vi "output.vi"(8 "error in":errorcluster, 10 "data table in":T1, 11 "SystemLin Tag Module runtime in":refnum<class "SystemLink runtime.lvclass">) -> (0 "error out":errorcluster, 2 "data table out":T1, 3 "SystemLin Tag Module runtime out":refnum<class "SystemLink runtime.lvclass">)   [LabVIEW 2014, in "SystemLink runtime.lvclass"]
doc: "Provides an interface for writing data to a module at runtime. While this interface performs no operations, a child should provide an override which may write to any open sessions, references, or interfaces."
uses:
  SystemLink runtime.lvclass
  <vilib>/NI/Tag Bus/table/data table.ctl
  SystemLink runtime.lvclass/SystemLink runtime.ctl
  <vilib>/NI/Tag Bus/table/data polymorphs/read one/read Double.vi
  <vilib>/NI/Tag Bus/table/data polymorphs/read one/read Single.vi
  <vilib>/NI/Tag Bus/table/data polymorphs/read one/read I32.vi
  <vilib>/NI/Tag Bus/table/data polymorphs/read one/read I16.vi
  <vilib>/NI/Tag Bus/table/data polymorphs/read one/read I8.vi
  <vilib>/NI/Tag Bus/table/data polymorphs/read one/read Boolean.vi
  <vilib>/NI/Tag Bus/table/data polymorphs/read one/read String.vi
  <vilib>/NI/Tag Bus/table/data table.lvlib
  <vilib>/Skyline/Tag/Wrapper/Wrapper_class/NI Skyline Tag.lvclass
  <vilib>/Skyline/Tag/Wrapper/Wrapper_class/Write Tag (DBL).vi
  <vilib>/Skyline/Tag/Wrapper/Wrapper_class/Write Tag (I32).vi
  <vilib>/Skyline/Tag/Wrapper/Wrapper_class/Write Tag (String).vi
  <vilib>/Skyline/Tag/Wrapper/Wrapper AMQP_class/NI Skyline Tag AMQP.lvclass
  <vilib>/Skyline/Tag/Wrapper/Wrapper HTTP_class/NI Skyline Tag HTTP.lvclass
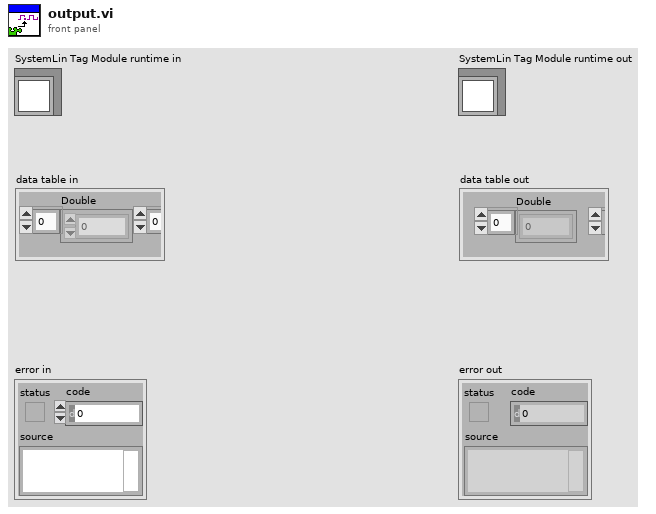
[diagram p1: front panel]
types:
  T1 = typedef "tag bus.lvlib/data table.lvlib/data table.ctl" = cluster{"Double":dbl[], "Single":sgl[], "I64":i64[], "I32":i32[], "I16":i16[], "I8":i8[], "U64":u64[], "U32":u32[], "U16":u16[], "U8":u8[], "Boolean":bool[], "String":string[], "Array of Double":cluster{"DBL Array":dbl[]}[], "Array of Single":cluster{"SGL Array":sgl[]}[], "Array of I64":cluster{"I64 Array":i64[]}[], "Array of I32":cluster{"I32 Array":i32[]}[], "Array of I16":cluster{"I16 Array":i16[]}[], "Array of I8":cluster{"I8 Array":i8[]}[], "Array of U64":cluster{"U64 Array":u64[]}[], "Array of U32":cluster{"U32 Array":u32[]}[], "Array of U16":cluster{"U16 Array":u16[]}[], "Array of U8":cluster{"U8 Array":u8[]}[], "Array of Boolean":cluster{"Boolean Array":bool[]}[], "Array of String":cluster{"String Array":string[]}[]}
  T2 = typedef "SystemLink configuration.lvclass/SysLink Mapping.ctl" = cluster{"Data Type":T3, "Tag Reference":refnum<class "NI Skyline Tag.lvclass">, "Tag Bus Index":i32, "AMQP":bool, "Skylink Index":i32}
  T3 = typedef "tag bus.lvlib/tag descriptor.lvclass/Data Type.ctl" = enum16{"Double", "Single", "I64", "I32", "I16", "I8", "U64", "U32", "U16", "U8", "Boolean", "String", "Array of Double", "Array of Single", "Array of I64", "Array of I32", "Array of I16", "Array of I8", "Array of U64", "Array of U32", "Array of U16", "Array of U8", "Array of Boolean", "Array of String"}
  T4 = typedef "NI Skyline Tag.lvlib/Tag Cluster Wrapper.ctl" = cluster{"Configuration":refnum<class "NI Skyline Configuration.lvclass">, "Tag Cluster":T5}
  T5 = typedef "NI Skyline Tag.lvlib/Tag Cluster.ctl" = cluster{"Path":string, "Data Type":T6, "Value":variant, "Time Stamp":timestamp}
  T6 = typedef "NI Skyline Tag.lvlib/DataType.ctl" = enum32{"Double", "Integer", "String"}
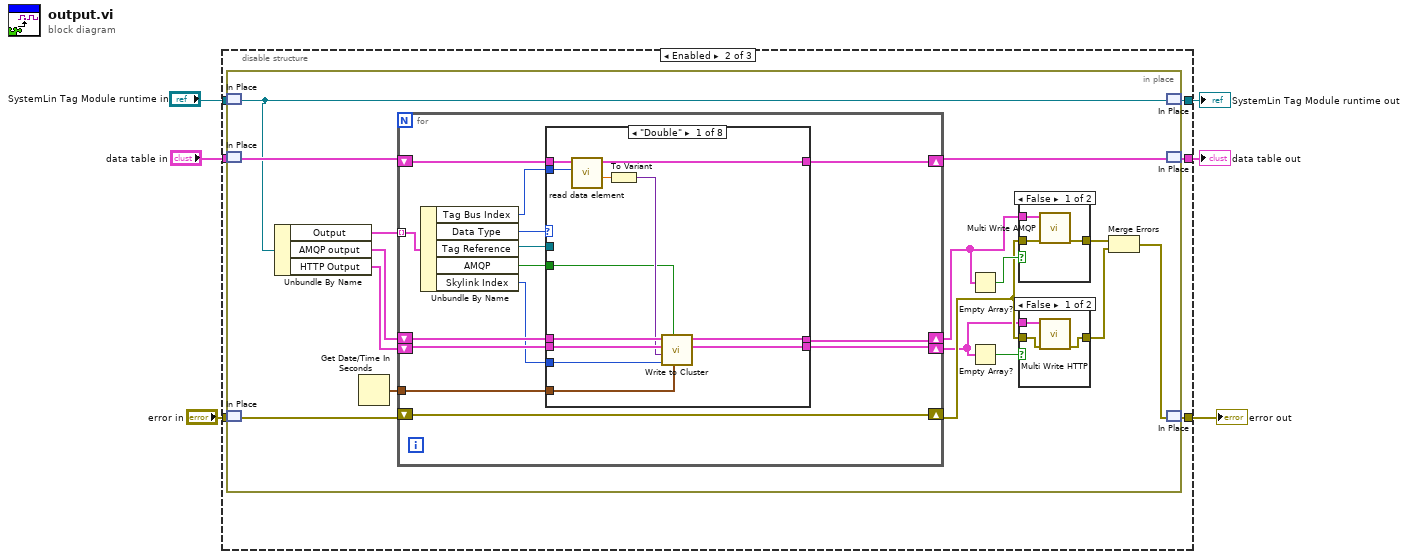
[diagram p0: block diagram]
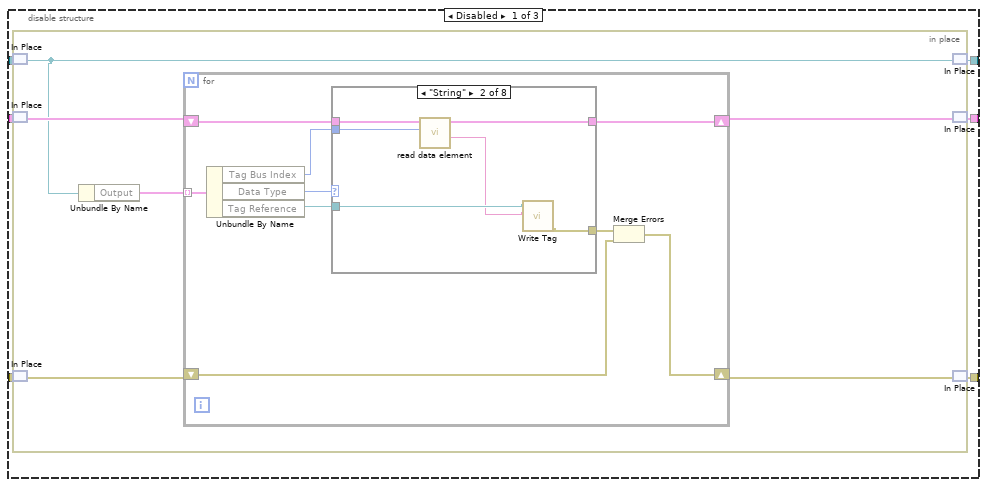
[diagram p2: hidden frame]
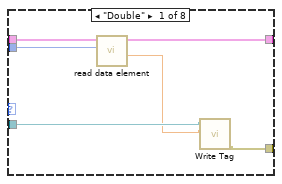
[diagram p3: hidden frame]
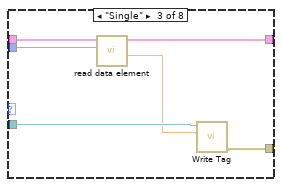
[diagram p4: hidden frame]
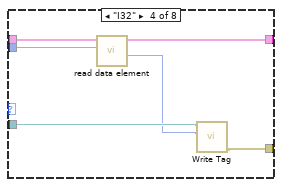
[diagram p5: hidden frame]
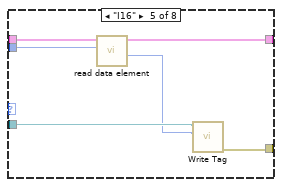
[diagram p6: hidden frame]
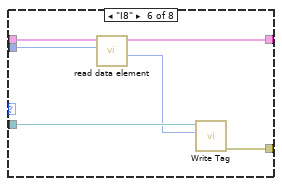
[diagram p7: hidden frame]
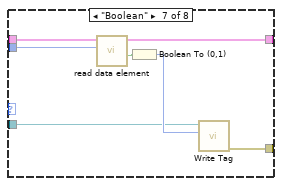
[diagram p8: hidden frame]
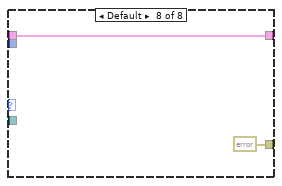
[diagram p9: hidden frame]
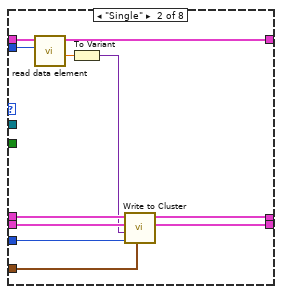
[diagram p12: hidden frame]
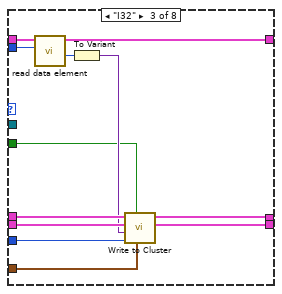
[diagram p13: hidden frame]
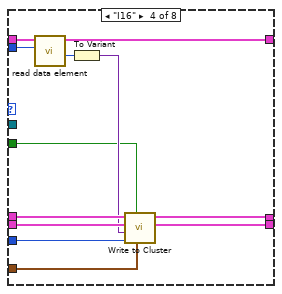
[diagram p14: hidden frame]
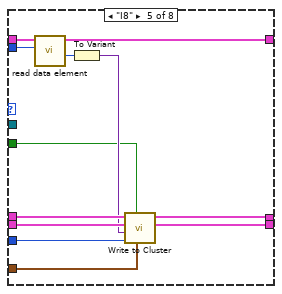
[diagram p15: hidden frame]
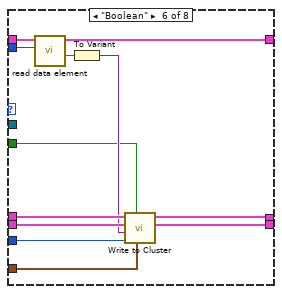
[diagram p16: hidden frame]
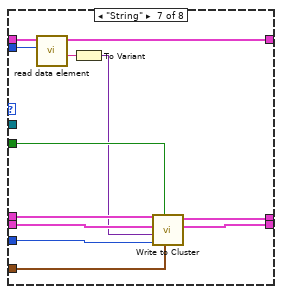
[diagram p17: hidden frame]
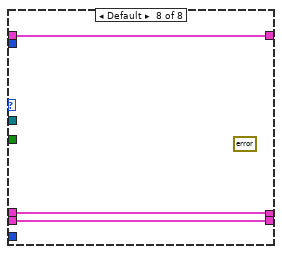
[diagram p18: hidden frame]
diagram:
  n1 = disable-structure shown="Enabled" {
    disable-tunnel: "SystemLin Tag Module runtime in" -> [w12 w78 _]
    disable-tunnel: [w11 w77 _] -> w5
    disable-tunnel: [w10 w76 _] -> w4
    disable-tunnel: [w9 w75 _] -> w3
    disable-tunnel: "data table in" -> [w8 w74 _]
    disable-tunnel: "error in" -> [w7 w73 _]
    frame Disabled {
      n2 = in-place {
        n3 = in-place-match #1(w12) -> (w16:refnum<class "SystemLink runtime.lvclass">)
        n4 = in-place-match #2(w8) -> (w18:T1)
        n5 = in-place-match #3(w7) -> (w14:errorcluster)
        n6 = Unbundle By Name(w16) -> ("Output"=w15:T2[])
        n7 = for {
          shift-right: [w24] -> w17
          shift-left: w18 -> [w25]
          tunnel: w15 -> [w27] mode=indexing
          shift-right: [w19] -> w13
          shift-left: w14 -> [w20]
          n8 = Unbundle By Name(w27) -> ("Tag Bus Index"=w22:i32, "Data Type"=w26:T3, "Tag Reference"=w23:refnum<class "NI Skyline Tag.lvclass">)
          n9 = case shown="\"String\"" w26 {
            tunnel: w25 -> [w33 w39 w45 w51 w57 w63 w70 w72]
            tunnel: [w31 w37 w43 w49 w55 w61 w68 w72] -> w24
            tunnel: w23 -> [w30 w36 w42 w48 w54 w60 w64 _]
            tunnel: [w28 w34 w40 w46 w52 w58 w67 errorcluster {"status"=FALSE, "code"=0, "source"=""} ("error IO")] -> w21
            tunnel: w22 -> [w32 w38 w44 w50 w56 w62 w69 _]
            frame "Double" {
              n10 = call-poly <vilib>:"read data element.vi"("index"=w32, "data table in"=w33) -> ("value"=w29:dbl, "data table out"=w31:T1)  [unwired: 8 in]
              n11 = call-poly <vilib>:"Write Tag.vi"("value"=w29, "tag in"=w30) -> ("error out"=w28:errorcluster)  [unwired: 8 in, 1 out]
            }
            frame "String" {
              n12 = call-poly <vilib>:"read data element.vi"("index"=w38, "data table in"=w39) -> ("value"=w35:string, "data table out"=w37:T1)  [unwired: 8 in]
              n13 = call-poly <vilib>:"Write Tag.vi"("value"=w35, "tag in"=w36) -> ("error out"=w34:errorcluster)  [unwired: 8 in, 1 out]
            }
            frame "Single" {
              n14 = call-poly <vilib>:"read data element.vi"("index"=w44, "data table in"=w45) -> ("value"=w41:sgl, "data table out"=w43:T1)  [unwired: 8 in]
              n15 = call-poly <vilib>:"Write Tag.vi"("value"=w41, "tag in"=w42) -> ("error out"=w40:errorcluster)  [unwired: 8 in, 1 out]
            }
            frame "I32" {
              n16 = call-poly <vilib>:"read data element.vi"("index"=w50, "data table in"=w51) -> ("value"=w47:i32, "data table out"=w49:T1)  [unwired: 8 in]
              n17 = call-poly <vilib>:"Write Tag.vi"("value"=w47, "tag in"=w48) -> ("error out"=w46:errorcluster)  [unwired: 8 in, 1 out]
            }
            frame "I16" {
              n18 = call-poly <vilib>:"read data element.vi"("index"=w56, "data table in"=w57) -> ("value"=w53:i16, "data table out"=w55:T1)  [unwired: 8 in]
              n19 = call-poly <vilib>:"Write Tag.vi"("value"=w53, "tag in"=w54) -> ("error out"=w52:errorcluster)  [unwired: 8 in, 1 out]
            }
            frame "I8" {
              n20 = call-poly <vilib>:"read data element.vi"("index"=w62, "data table in"=w63) -> ("value"=w59:i8, "data table out"=w61:T1)  [unwired: 8 in]
              n21 = call-poly <vilib>:"Write Tag.vi"("value"=w59, "tag in"=w60) -> ("error out"=w58:errorcluster)  [unwired: 8 in, 1 out]
            }
            frame "Boolean" {
              n22 = call-poly <vilib>:"read data element.vi"("index"=w69, "data table in"=w70) -> ("value"=w65:bool, "data table out"=w68:T1)  [unwired: 8 in]
              n23 = Boolean To (0,1)(Boolean=w65) -> (0, 1=w66:i16)
              n24 = call-poly <vilib>:"Write Tag.vi"("value"=w66, "tag in"=w64) -> ("error out"=w67:errorcluster)  [unwired: 8 in, 1 out]
            }
            frame Default {
            }
          }
          n25 = Merge Errors(w21, w20) -> (w19:errorcluster)
        }
        n26 = in-place-match #1(w16) -> (w11:refnum<class "SystemLink runtime.lvclass">)
        n27 = in-place-match #2(w17) -> (w10:T1)
        n28 = in-place-match #3(w13) -> (w9:errorcluster)
      }
    }
    frame Enabled {
      n29 = in-place {
        n30 = in-place-match #4(w78) -> (w92:refnum<class "SystemLink runtime.lvclass">)
        n31 = in-place-match #5(w74) -> (w94:T1)
        n32 = in-place-match #6(w73) -> (w90:errorcluster)
        n33 = Unbundle By Name(w92) -> ("Output"=w91:T2[], "AMQP output"=w89:T4[], "HTTP Output"=w88:T4[])
        n34 = Get Date/Time In Seconds() -> (seconds since 1Jan1904=w79:timestamp)
        n35 = for {
          shift-right: [w113] -> w93
          shift-left: w94 -> [w114]
          tunnel: w91 -> [w116] mode=indexing
          shift-right: [w110] -> w83
          shift-left: w90 -> [w110]
          shift-right: [w104] -> w81
          shift-left: w88 -> [w108]
          shift-right: [w105] -> w80
          shift-left: w89 -> [w109]
          tunnel: w79 -> [w103]
          n36 = Unbundle By Name(w116) -> ("Tag Bus Index"=w111:i32, "Data Type"=w115:T3, "Tag Reference"=w112:refnum<class "NI Skyline Tag.lvclass">, "AMQP"=w107:bool, "Skylink Index"=w106:i32)
          n37 = case shown="\"Double\"" w115 {
            tunnel: w114 -> [w128 w139 w151 w163 w175 w187 w199 w202]
            tunnel: [w126 w137 w149 w161 w173 w185 w197 w202] -> w113
            tunnel: w112 -> [_ _ _ _ _ _ _ _]
            tunnel: w111 -> [w127 w138 w150 w162 w174 w186 w198 _]
            tunnel: w109 -> [w125 w136 w148 w160 w172 w184 w194 w201]
            tunnel: w108 -> [w124 w135 w147 w159 w171 w183 w193 w200]
            tunnel: w107 -> [w117 _ w140 w152 w164 w176 w192 _]
            tunnel: w106 -> [w120 w131 w143 w155 w167 w179 w189 _]
            tunnel: [w123 w134 w146 w158 w170 w182 w196 w201] -> w105
            tunnel: [w122 w133 w145 w157 w169 w181 w195 w200] -> w104
            tunnel: w103 -> [w121 w132 w144 w156 w168 w180 w191 _]
            frame "Double" {
              n38 = call-poly <vilib>:"read data element.vi"("index"=w127, "data table in"=w128) -> ("value"=w119:dbl, "data table out"=w126:T1)  [unwired: 8 in]
              n39 = To Variant(anything=w119) -> (Variant=w118:variant)
              n40 = call "Write to Cluster.vi"("Tag Cluster.Time Stamp"=w121, "AMQP"=w117, "Skylink Index"=w120, "Variant"=w118, "HTTP  in"=w124, "AMQP  in"=w125) -> ("HTTP  out"=w122:T4[], "AMQP  out"=w123:T4[])  [unwired: 4 in]
            }
            frame "Single" {
              n41 = call-poly <vilib>:"read data element.vi"("index"=w138, "data table in"=w139) -> ("value"=w130:sgl, "data table out"=w137:T1)  [unwired: 8 in]
              n42 = To Variant(anything=w130) -> (Variant=w129:variant)
              n43 = call "Write to Cluster.vi"("Tag Cluster.Time Stamp"=w132, "Skylink Index"=w131, "Variant"=w129, "HTTP  in"=w135, "AMQP  in"=w136) -> ("HTTP  out"=w133:T4[], "AMQP  out"=w134:T4[])  [unwired: 5 in]
            }
            frame "I32" {
              n44 = call-poly <vilib>:"read data element.vi"("index"=w150, "data table in"=w151) -> ("value"=w142:i32, "data table out"=w149:T1)  [unwired: 8 in]
              n45 = To Variant(anything=w142) -> (Variant=w141:variant)
              n46 = call "Write to Cluster.vi"("Tag Cluster.Time Stamp"=w144, "AMQP"=w140, "Skylink Index"=w143, "Variant"=w141, "HTTP  in"=w147, "AMQP  in"=w148) -> ("HTTP  out"=w145:T4[], "AMQP  out"=w146:T4[])  [unwired: 4 in]
            }
            frame "I16" {
              n47 = call-poly <vilib>:"read data element.vi"("index"=w162, "data table in"=w163) -> ("value"=w154:i16, "data table out"=w161:T1)  [unwired: 8 in]
              n48 = To Variant(anything=w154) -> (Variant=w153:variant)
              n49 = call "Write to Cluster.vi"("Tag Cluster.Time Stamp"=w156, "AMQP"=w152, "Skylink Index"=w155, "Variant"=w153, "HTTP  in"=w159, "AMQP  in"=w160) -> ("HTTP  out"=w157:T4[], "AMQP  out"=w158:T4[])  [unwired: 4 in]
            }
            frame "I8" {
              n50 = call-poly <vilib>:"read data element.vi"("index"=w174, "data table in"=w175) -> ("value"=w166:i8, "data table out"=w173:T1)  [unwired: 8 in]
              n51 = To Variant(anything=w166) -> (Variant=w165:variant)
              n52 = call "Write to Cluster.vi"("Tag Cluster.Time Stamp"=w168, "AMQP"=w164, "Skylink Index"=w167, "Variant"=w165, "HTTP  in"=w171, "AMQP  in"=w172) -> ("HTTP  out"=w169:T4[], "AMQP  out"=w170:T4[])  [unwired: 4 in]
            }
            frame "Boolean" {
              n53 = call-poly <vilib>:"read data element.vi"("index"=w186, "data table in"=w187) -> ("value"=w178:bool, "data table out"=w185:T1)  [unwired: 8 in]
              n54 = To Variant(anything=w178) -> (Variant=w177:variant)
              n55 = call "Write to Cluster.vi"("Tag Cluster.Time Stamp"=w180, "AMQP"=w176, "Skylink Index"=w179, "Variant"=w177, "HTTP  in"=w183, "AMQP  in"=w184) -> ("HTTP  out"=w181:T4[], "AMQP  out"=w182:T4[])  [unwired: 4 in]
            }
            frame "String" {
              n56 = call-poly <vilib>:"read data element.vi"("index"=w198, "data table in"=w199) -> ("value"=w188:string, "data table out"=w197:T1)  [unwired: 8 in]
              n57 = To Variant(anything=w188) -> (Variant=w190:variant)
              n58 = call "Write to Cluster.vi"("Tag Cluster.Time Stamp"=w191, "AMQP"=w192, "Skylink Index"=w189, "Variant"=w190, "HTTP  in"=w193, "AMQP  in"=w194) -> ("HTTP  out"=w195:T4[], "AMQP  out"=w196:T4[])  [unwired: 4 in]
            }
            frame Default {
              (unwired) errorcluster {"status"=FALSE, "code"=0, "source"=""} ("error IO")
            }
          }
        }
        n59 = Empty Array?(array=w80) -> (empty?=w86:bool)
        n60 = Empty Array?(array=w81) -> (empty?=w87:bool)
        n61 = case shown="False" w86 {
          tunnel: [w101 w102] -> w85
          tunnel: w80 -> [w100 _]
          tunnel: w83 -> [w99 w102]
          frame False {
            n62 = call <vilib>:"Multi Write AMQP.vi"("error in (no error)"=w99, "tags in"=w100) -> ("error out"=w101:errorcluster)  [unwired: 9 in]
          }
          frame True {
          }
        }
        n63 = case shown="False" w87 {
          tunnel: [w97 w98] -> w84
          tunnel: w81 -> [w96 _]
          tunnel: w83 -> [w95 w98]
          frame False {
            n64 = call <vilib>:"Multi Write HTTP.vi"("error in (no error)"=w95, "tag clusters"=w96) -> ("error out"=w97:errorcluster)  [unwired: 9 in]
          }
          frame True {
          }
        }
        n65 = Merge Errors(w85, w84) -> (w82:errorcluster)
        n66 = in-place-match #4(w92) -> (w77:refnum<class "SystemLink runtime.lvclass">)
        n67 = in-place-match #5(w93) -> (w76:T1)
        n68 = in-place-match #6(w82) -> (w75:errorcluster)
      }
    }
    frame Disabled {
    }
  }
  "error out" <- w3
  "SystemLin Tag Module runtime out" <- w5
  "data table out" <- w4
